vi "MovingAverage.vi"(3 "error in":errorcluster, 4 "Points to average":i32=200, 5 "Input array":dbl[](array[numeric])) -> (0 "error out":errorcluster, 2 "Output array":dbl[](array[numeric]))   [LabVIEW 2015]
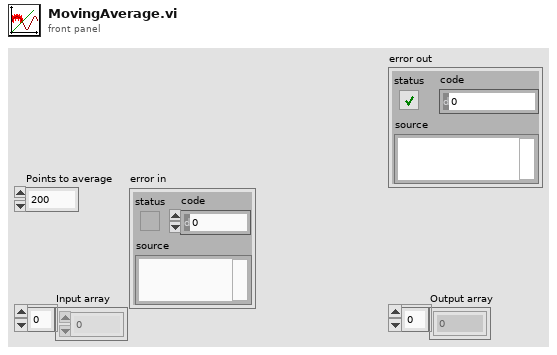
[diagram p1: front panel]
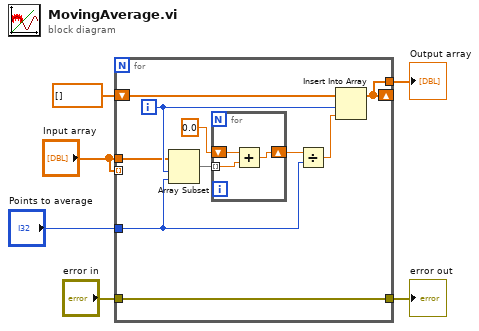
[diagram p0: block diagram]
diagram:
  n1 = for {
    tunnel: [w11] -> w5
    shift-right: [w11] -> _
    shift-left: dbl[] [] -> [w10]
    tunnel: "Input array" -> [_] mode=indexing
    tunnel: "Input array" -> [w9]
    tunnel: "Points to average" -> [w8]
    tunnel: "error in" -> [w7]
    tunnel: [w7] -> w1
    i -> [w13]
    n2 = Array Subset(array=w9, index=w13, length=w8) -> (w16:dbl[])
    n3 = for {
      tunnel: w16 -> [w17] mode=indexing
      shift-right: [w19] -> w14
      shift-left: 0.0 -> [w18]
      n4 = Add(x=w18, y=w17) -> (x+y=w19:dbl)
    }
    n5 = Divide(x=w14, y=w8) -> (x/y=w12:dbl)
    n6 = Insert Into Array(array=w10, index=w13, new element=w12) -> (w11:dbl[])
  }
  "Output array" <- w5
  "error out" <- w1
